vi "ProcessName.vi"() -> (1 "process name":string)   [LabVIEW 2017, in "IrAnalysis.lvlib"]
uses:
  <vilib>/addons/InsightCM/Devices/Shared/Ir/IrAnalysis/IrAnalysis.lvlib
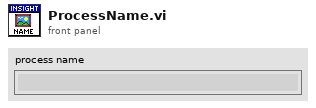
[diagram p1: front panel]
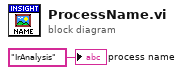
[diagram p0: block diagram]
diagram:
  "process name" <- "IrAnalysis" ("ProcessName")
